vi "Free-libraries.vi"(8 "error in (no error)":errorcluster, 11 "SM1000-control in":T1) -> (0 "error out":errorcluster, 1 "Loaded?":bool, 3 "SM1000-control out":T1)   [LabVIEW 2013, in "HardwareCharacterization.lvlib" / "HC-SM1000.lvclass"]
uses:
  HC-SM1000.lvclass
  Object-reference.ctl
  HC-SM1000.lvclass/HC-SM1000.ctl
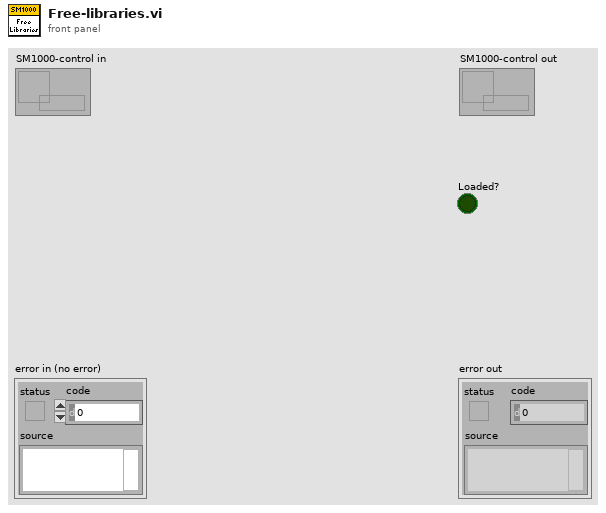
[diagram p1: front panel]
types:
  T1 = typedef "HardwareCharacterization.lvlib/HC-SM1000.lvclass/Object-reference.ctl" = refnum<data-value>
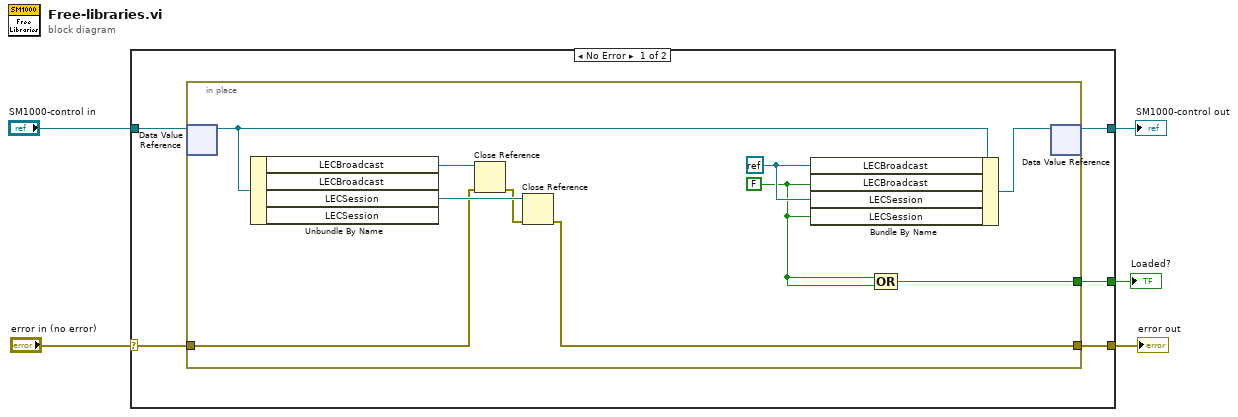
[diagram p0: block diagram]
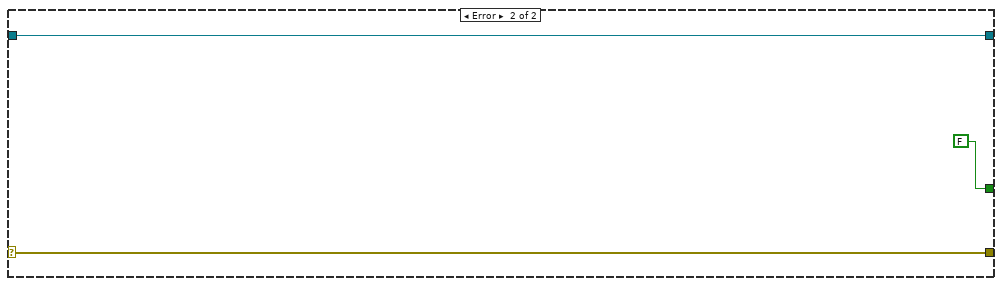
[diagram p2: hidden frame]
diagram:
  n1 = case shown="No Error" "error in (no error)" {
    selector: "error in (no error)" -> [w8 w23]
    tunnel: [w6 w23] -> w4
    tunnel: [w9 w22] -> w2
    tunnel: "SM1000-control in" -> [w10 w22]
    tunnel: [w7 FALSE] -> w1
    frame No Error {
      n2 = in-place {
        in-place-border: w8 -> [w13]
        in-place-border: [w19] -> w7
        in-place-border: [w11] -> w6
        w14 = FALSE
        w15 = refnum<k0> refnum
        n3 = in-place-dvr #1(w10) -> (w18:refnum<class "HC-SM1000.lvclass">)  [unwired: 1 out]
        n4 = Unbundle By Name(w18) -> ("LECBroadcast"=w17:refnum<k24>, "LECSession"=w16:refnum<k24>)  [unwired: 2 out]
        n5 = Close Reference(reference=w17, error in (no error)=w13) -> (error out=w12:errorcluster)
        n6 = Close Reference(reference=w16, error in (no error)=w12) -> (error out=w11:errorcluster)
        n7 = Bundle By Name(cluster=w18, "LECBroadcast"=w15, "LECBroadcast"=w14, "LECSession"=w15, "LECSession"=w14) -> (w20:refnum<class "HC-SM1000.lvclass">)
        n8 = Compound Arithmetic op=OR(w14, w14) -> (w19:bool)
        n9 = in-place-dvr #1(w20) -> (w9:T1)  [unwired: 1 out]
      }
    }
    frame Error {
    }
  }
  "error out" <- w4
  "SM1000-control out" <- w2
  "Loaded?" <- w1
